vi "hw2-2 topVI.vi"() -> ()   [LabVIEW 2014]
panel:
  out "Array":dbl[](array[numeric])
  out "Sorted Array":dbl[](array[numeric])
  out "swap":bool
  out "XY Graph":cluster{i32[], dbl[]}(graph)
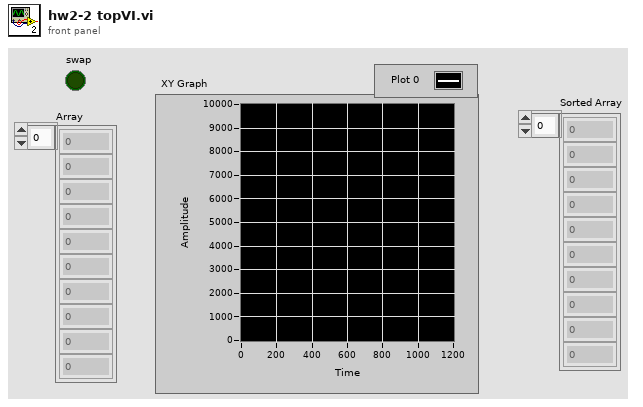
[diagram p1: front panel]
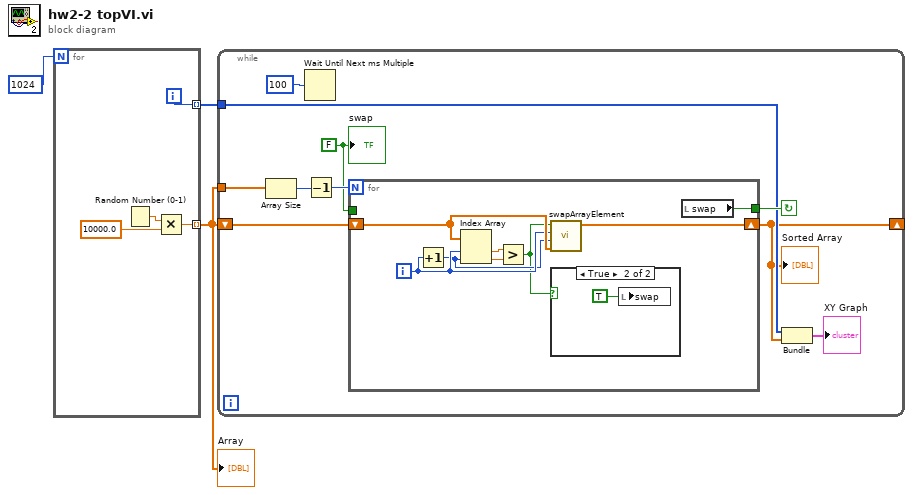
[diagram p0: block diagram]
diagram:
  n1 = for {
    N: 1024 -> [_]
    tunnel: [w5] -> w2 mode=indexing
    tunnel: [w4] -> w1 mode=indexing
    i -> [w4]
    n2 = Random Number (0-1)() -> (number: 0 to 1=w7:dbl)
    n3 = Multiply(x=w7, y=10000.0) -> (x*y=w5:dbl)
  }
  "Array" <- w2
  n4 = while {
    tunnel: w2 -> [w14]
    shift-right: [w9] -> _
    shift-left: w2 -> [w13]
    tunnel: w1 -> [w10]
    stop <- w12 continue-if-true
    w15 = FALSE
    n5 = Array Size(array=w14) -> (size(s)=w17:i32)
    n6 = Wait Until Next ms Multiple(millisecond multiple=u32 100) -> ()  [unwired: 1 out]
    n7 = Decrement(x=w17) -> (x-1=w16:i32)
    n8 = for {
      N: w16 -> [_]
      shift-right: [w19] -> w9
      shift-left: w13 -> [w22]
      tunnel: w15 -> [_]
      tunnel: [w23] -> w12
      i -> [w21]
      n9 = Increment(x=w21) -> (x+1=w20:i32)
      n10 = Index Array(array=w22, index #1=w21, index #2=w20) -> (element #1=w25:dbl, element #2=w24:dbl)
      n11 = Greater?(x=w25, y=w24) -> (0:w18:bool)
      n12 = call "swapArrayElement.vi"("Array"=w22, "Index 2"=w20, "Index 1"=w21, "swap"=w18) -> ("Swapped Array"=w19:dbl[])  [unwired: 7 in]
      n13 = case shown="True" w18 {
        frame False {
        }
        frame True {
          n14 = local write "swap"(TRUE) -> ()
        }
      }
      n15 = local read "swap"() -> (w23:bool)
    }
    "Sorted Array" <- w9
    n16 = Bundle(w10, w9) -> (→"XY Graph":cluster{i32[], dbl[]})  [unwired: 1 in]
    "swap" <- w15
  }
